vi "station1_bit to array.vi"(8 "error in (no error)":errorcluster, 11 "ST1_Controls_from_PLC":i64[](array[numeric])=[0, 0, 0, 0, 0]) -> (0 "error out":errorcluster, 2 "1 on state":i32[](array[numeric]), 3 "1 result array":bool[](array[boolean]))   [LabVIEW 2017]
panel:
  out "fpl st1":bool
  out "cycle rslt":bool
  out "cycle status":bool
  out "driver st1":bool
  out "LB st1":bool
  out "HB st1":bool
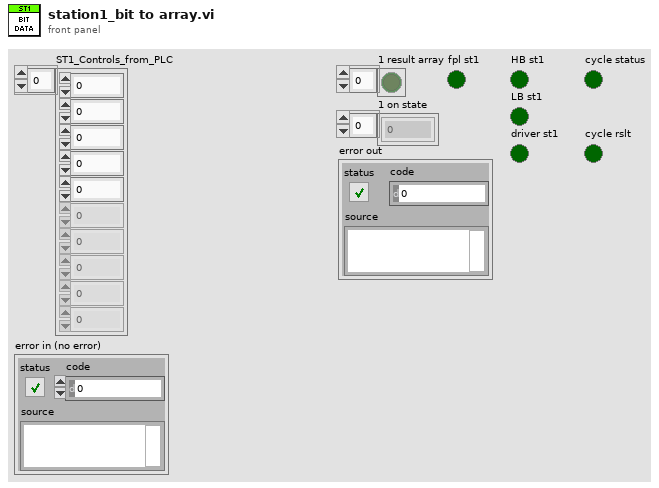
[diagram p1: front panel]
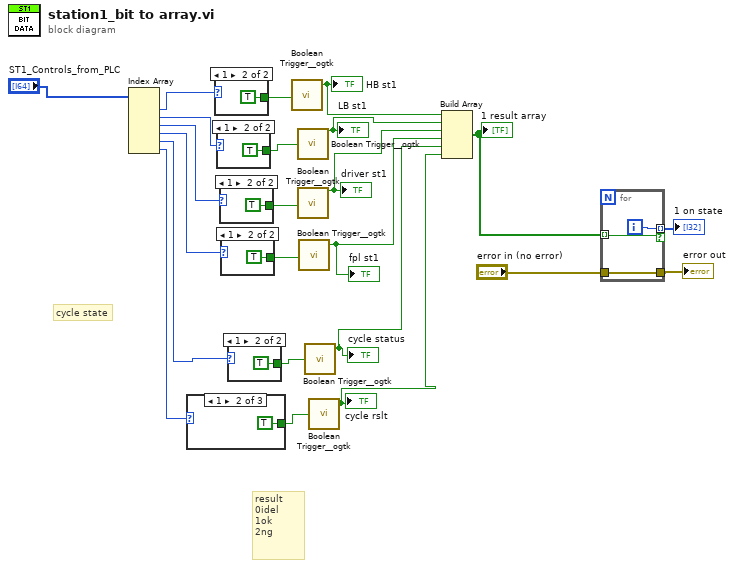
[diagram p0: block diagram]
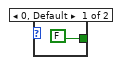
[diagram p2: hidden frame]
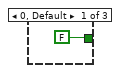
[diagram p3: hidden frame]
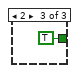
[diagram p4: hidden frame]
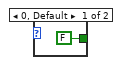
[diagram p5: hidden frame]
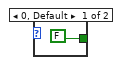
[diagram p6: hidden frame]
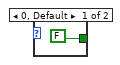
[diagram p7: hidden frame]
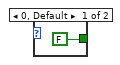
[diagram p8: hidden frame]
diagram:
  # "cycle state"
  # "result\n0idel\n1ok\n2ng"
  n1 = Index Array(array="ST1_Controls_from_PLC") -> (element #1=w23:i64, element #2=w22:i64, element #3=w21:i64, element #4=w3:i64, element #5=w2:i64, element #6=w1:i64)  [unwired: 6 in]
  n2 = case shown="1" w1 {
    tunnel: [FALSE TRUE TRUE] -> w19
    frame 0, Default {
    }
    frame 1 {
    }
    frame 2 {
    }
  }
  n3 = case shown="1" w23 {
    tunnel: [FALSE TRUE] -> w16
    frame 0, Default {
    }
    frame 1 {
    }
  }
  n4 = case shown="1" w22 {
    tunnel: [FALSE TRUE] -> w17
    frame 0, Default {
    }
    frame 1 {
    }
  }
  n5 = case shown="1" w21 {
    tunnel: [FALSE TRUE] -> w18
    frame 0, Default {
    }
    frame 1 {
    }
  }
  n6 = case shown="1" w3 {
    tunnel: [FALSE TRUE] -> w7
    frame 0, Default {
    }
    frame 1 {
    }
  }
  n7 = case shown="1" w2 {
    tunnel: [FALSE TRUE] -> w20
    frame 0, Default {
    }
    frame 1 {
    }
  }
  n8 = call <userlib>:"Boolean Trigger__ogtk.vi"("Boolean Input"=w16) -> ("Rising Edge"=w14:bool)  [unwired: 1 in, 1 out]
  "HB st1" <- w14
  n9 = call <userlib>:"Boolean Trigger__ogtk.vi"("Boolean Input"=w17) -> ("Rising Edge"=w13:bool)  [unwired: 1 in, 1 out]
  "LB st1" <- w13
  n10 = call <userlib>:"Boolean Trigger__ogtk.vi"("Boolean Input"=w18) -> ("Rising Edge"=w12:bool)  [unwired: 1 in, 1 out]
  "driver st1" <- w12
  n11 = call <userlib>:"Boolean Trigger__ogtk.vi"("Boolean Input"=w7) -> ("Rising Edge"=w4:bool)  [unwired: 1 in, 1 out]
  "fpl st1" <- w4
  n12 = call <userlib>:"Boolean Trigger__ogtk.vi"("Boolean Input"=w20) -> ("Rising Edge"=w6:bool)  [unwired: 1 in, 1 out]
  "cycle status" <- w6
  n13 = call <userlib>:"Boolean Trigger__ogtk.vi"("Boolean Input"=w19) -> ("Rising Edge"=w5:bool)  [unwired: 1 in, 1 out]
  "cycle rslt" <- w5
  n14 = Build Array(w14, w13, w12, w4, w6, w5) -> (w11:bool[])
  "1 result array" <- w11
  n15 = for {
    tunnel: [w39] -> w10 mode=indexing if=w37
    tunnel: "error in (no error)" -> [w38]
    tunnel: [w38] -> w9
    tunnel: w11 -> [w37] mode=indexing
    i -> [w39]
  }
  "1 on state" <- w10
  "error out" <- w9
